vi "Supply Line Config.vi"(0 "Supply Line Handle in":refnum<k15>, 5 "SMU Config":T1={"Output Function"=1006, "Channel(s)"="", "Voltage Level"=0.0, "Current Level"=0.0, "Voltage Limit"=0.0, "Current Limit"=0.0, "Transient Response (V):Gain Bandwidth"=0.0, "Transient Response (V):Compensation Frequency"=0.0, "Transient Response (V):Pole-Zero Ratio"=0.0, "Transient Response"=1039, "Sense"=1009, "Transient Response (I):Gain Bandwidth"=0.0, "Transient Response (I):Compensation Frequency"=0.0, "Transient Response (I):Pole-Zero Ratio"=0.0} {"Sense" items=["Local"=1008, "Remote"=1009]; "Transient Response" items=["Slow"=1041, "Normal"=1038, "Fast"=1039, "Custom"=1042]; "output function" items=["DC Voltage"=1006, "DC Current"=1007, "Pulse Voltage"=1049, "Pulse Current"=1050]}, 11 "error in (no error)":errorcluster) -> (4 "Supply Line Handle out":refnum<k15>, 15 "error out":errorcluster)   [LabVIEW 2016, in "SMU.lvlib"]
uses:
  SMU.lvlib
  <instrlib>/niDCPower/nidcpower.llb/niDCPower Source Mode.ctl
  <instrlib>/niDCPower/nidcpower.llb/niDCPower Output Function.ctl
  Typedefs/Supply Line Configuration.ctl
panel:
  out "Source:Custom Transient Response:Current:Gain Bandwidth":dbl
  out "Source:Custom Transient Response:Current:Compensation Frequency":dbl
  out "Source:Custom Transient Response:Current:Pole-Zero Ratio":dbl
  out "Source:Custom Transient Response:Voltage:Pole-Zero Ratio":dbl
  out "Source:Custom Transient Response:Voltage:Compensation Frequency":dbl
  out "Source:Custom Transient Response:Voltage:Gain Bandwidth":dbl
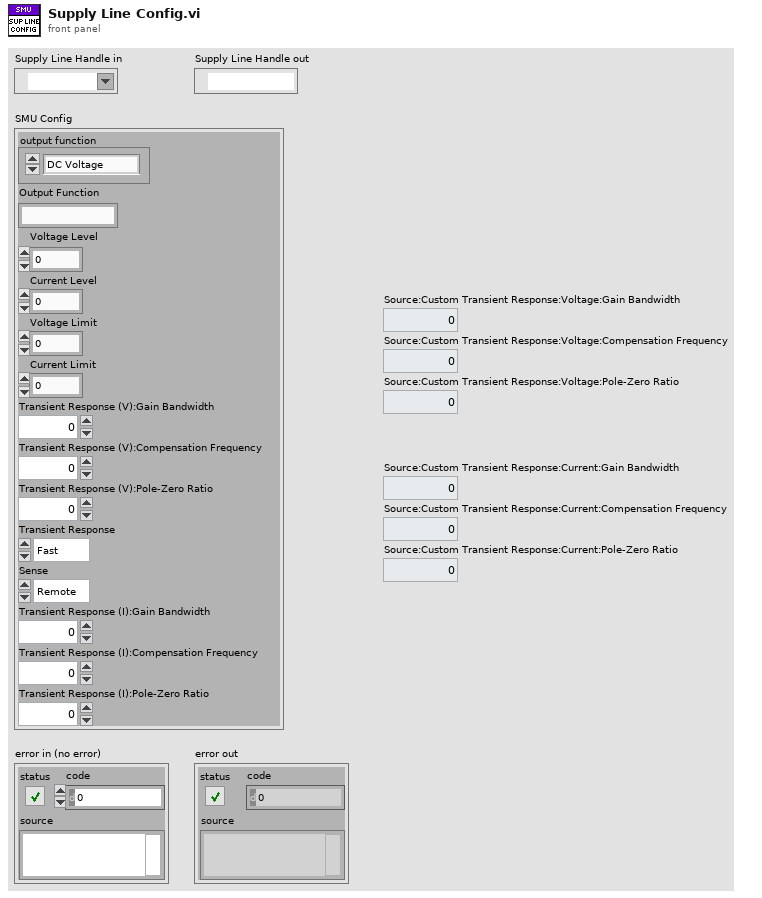
[diagram p1: front panel]
types:
  T1 = typedef "SMU.lvlib/Supply Line Configuration.ctl" = cluster{"Output Function":T2, "Channel(s)":string, "Voltage Level":dbl, "Current Level":dbl, "Voltage Limit":dbl, "Current Limit":dbl, "Transient Response (V):Gain Bandwidth":dbl, "Transient Response (V):Compensation Frequency":dbl, "Transient Response (V):Pole-Zero Ratio":dbl, "Transient Response":i32, "Sense":i32, "Transient Response (I):Gain Bandwidth":dbl, "Transient Response (I):Compensation Frequency":dbl, "Transient Response (I):Pole-Zero Ratio":dbl}
  T2 = typedef "niDCPower Output Function.ctl" = i32
  T3 = typedef "niDCPower Source Mode.ctl" = i32
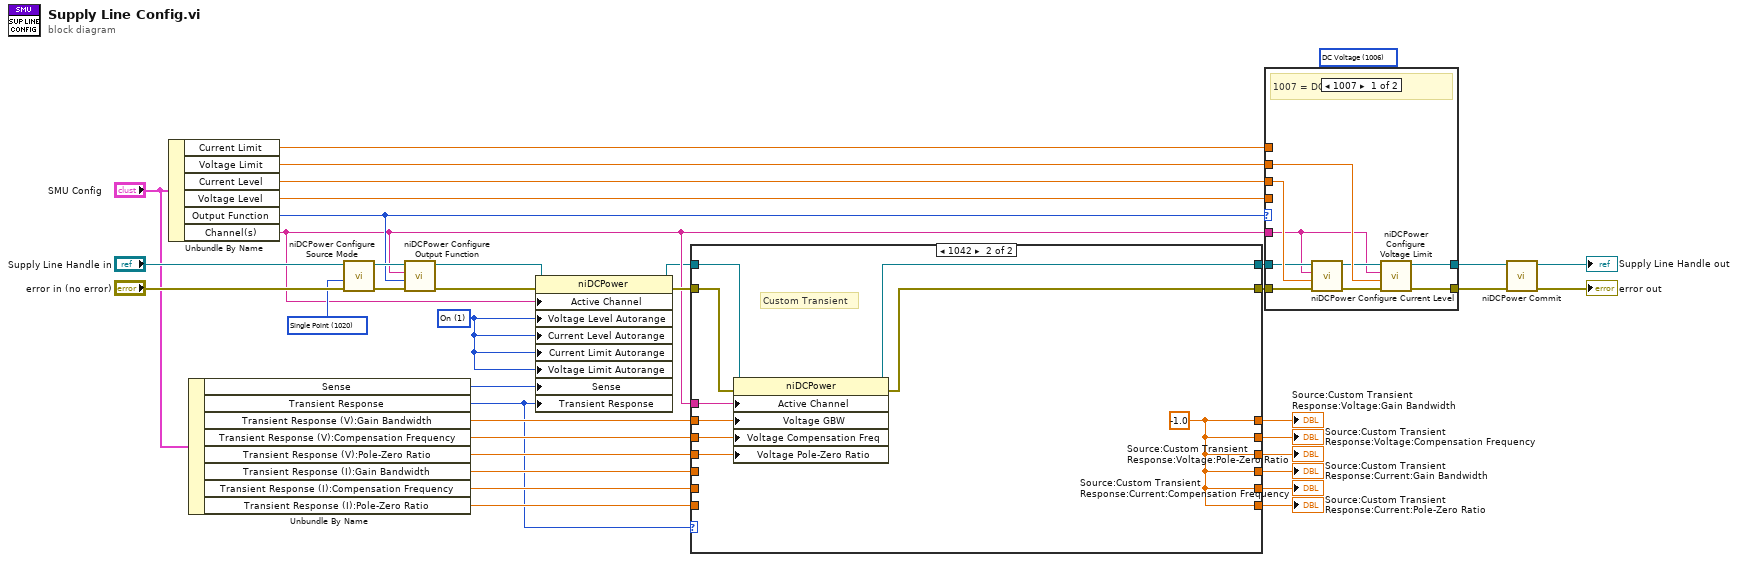
[diagram p0: block diagram]
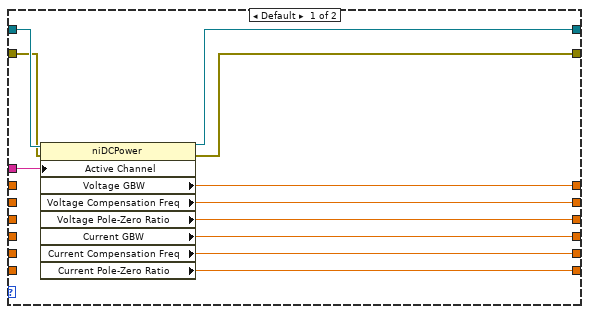
[diagram p2: hidden frame]
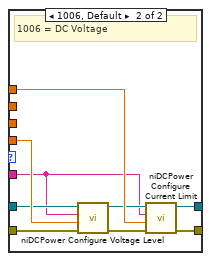
[diagram p3: hidden frame]
diagram:
  w20 = 1 items=["Off", "On"] ("Source:DC Voltage:Voltage Level Autorange")
  (unwired) T2 1006 items=["DC Voltage"=1006, "DC Current"=1007, "Pulse Voltage"=1049, "Pulse Current"=1050] ("Output Function")
  w31 = T3 1020 items=["Single Point"=1020, "Sequence"=1021] ("source mode")
  n1 = Unbundle By Name("SMU Config") -> ("Current Limit"=w28:dbl, "Voltage Limit"=w27:dbl, "Current Level"=w29:dbl, "Voltage Level"=w30:dbl, "Output Function"=w24:T2, "Channel(s)"=w17:string)
  n2 = Unbundle By Name("SMU Config") -> ("Sense"=w18:i32, "Transient Response"=w7:i32, "Transient Response (V):Gain Bandwidth"=w8:dbl, "Transient Response (V):Compensation Frequency"=w9:dbl, "Transient Response (V):Pole-Zero Ratio"=w10:dbl, "Transient Response (I):Gain Bandwidth"=w11:dbl, "Transient Response (I):Compensation Frequency"=w12:dbl, "Transient Response (I):Pole-Zero Ratio"=w13:dbl)
  n3 = call <instrlib>:"niDCPower Configure Source Mode.vi"("error in (no error)"="error in (no error)", "source mode"=w31, "instrument handle"="Supply Line Handle in") -> ("error out"=w37:errorcluster, "instrument handle out"=w25:refnum<k15>)  [unwired: 7 out]
  n4 = call <instrlib>:"niDCPower Configure Output Function.vi"("error in (no error)"=w37, "output function"=w24, "channel name"=w17, "instrument handle"=w25) -> ("error out"=w35:errorcluster, "instrument handle out"=w23:refnum<k15>)  [unwired: 6 in]
  n5 = property class="niDCPower"(reference=w23, error in=w35, "Active Channel"=w17, "Voltage Level Autorange"=w20, "Current Level Autorange"=w20, "Current Limit Autorange"=w20, "Voltage Limit Autorange"=w20, "Sense"=w18, "Transient Response"=w7) -> (reference out=w14:refnum<k15>, error out=w32:errorcluster)
  n6 = case shown="1042" w7 {
    tunnel: w32 -> [w44 w57]
    tunnel: w17 -> [w48 w56]
    tunnel: [w46 w55] -> w16
    tunnel: [w45 w54] -> w15
    tunnel: w14 -> [w47 w53]
    tunnel: w13 -> [_ _]
    tunnel: w12 -> [_ _]
    tunnel: w11 -> [_ _]
    tunnel: w10 -> [_ w52]
    tunnel: w9 -> [_ w51]
    tunnel: w8 -> [_ w50]
    tunnel: [w43 w49] -> w6
    tunnel: [w42 w49] -> w5
    tunnel: [w41 w49] -> w4
    tunnel: [w40 w49] -> w3
    tunnel: [w39 w49] -> w2
    tunnel: [w38 w49] -> w1
    frame Default {
      n7 = property class="niDCPower"(reference=w47, error in=w44, "Active Channel"=w48) -> (reference out=w46:refnum<k15>, error out=w45:errorcluster, "Voltage GBW"=w43:dbl, "Voltage Compensation Freq"=w42:dbl, "Voltage Pole-Zero Ratio"=w41:dbl, "Current GBW"=w40:dbl, "Current Compensation Freq"=w39:dbl, "Current Pole-Zero Ratio"=w38:dbl)
    }
    frame 1042 {
      w49 = -1.0 ("Voltage GBW")
      # "Custom Transient"
      n8 = property class="niDCPower"(reference=w53, error in=w57, "Active Channel"=w56, "Voltage GBW"=w50, "Voltage Compensation Freq"=w51, "Voltage Pole-Zero Ratio"=w52) -> (reference out=w55:refnum<k15>, error out=w54:errorcluster)
    }
  }
  "Source:Custom Transient Response:Voltage:Gain Bandwidth" <- w6
  "Source:Custom Transient Response:Voltage:Compensation Frequency" <- w5
  "Source:Custom Transient Response:Voltage:Pole-Zero Ratio" <- w4
  "Source:Custom Transient Response:Current:Gain Bandwidth" <- w3
  "Source:Custom Transient Response:Current:Compensation Frequency" <- w2
  "Source:Custom Transient Response:Current:Pole-Zero Ratio" <- w1
  n9 = case shown="1007" w24 {
    tunnel: [w63 w72] -> w22
    tunnel: w17 -> [w58 w67]
    tunnel: w30 -> [_ w71]
    tunnel: w29 -> [w62 _]
    tunnel: w28 -> [_ w70]
    tunnel: w27 -> [w61 _]
    tunnel: [w65 w74] -> w34
    tunnel: w16 -> [w59 w68]
    tunnel: w15 -> [w64 w73]
    frame 1007 {
      # "1007 = DC Current"
      n10 = call <instrlib>:"niDCPower Configure Current Level.vi"("error in (no error)"=w64, "current level"=w62, "channel name"=w58, "instrument handle"=w59) -> ("error out"=w66:errorcluster, "instrument handle out"=w60:refnum<k15>)  [unwired: 6 in]
      n11 = call <instrlib>:"niDCPower Configure Voltage Limit.vi"("error in (no error)"=w66, "voltage limit"=w61, "channel name"=w58, "instrument handle"=w60) -> ("error out"=w65:errorcluster, "instrument handle out"=w63:refnum<k15>)  [unwired: 6 in]
    }
    frame 1006, Default {
      # "1006 = DC Voltage"
      n12 = call <instrlib>:"niDCPower Configure Voltage Level.vi"("error in (no error)"=w73, "voltage level"=w71, "channel name"=w67, "instrument handle"=w68) -> ("error out"=w75:errorcluster, "instrument handle out"=w69:refnum<k15>)  [unwired: 6 out]
      n13 = call <instrlib>:"niDCPower Configure Current Limit.vi"("error in (no error)"=w75, "current limit"=w70, "channel name"=w67, "instrument handle"=w69) -> ("error out"=w74:errorcluster, "instrument handle out"=w72:refnum<k15>)  [unwired: 1 in, 5 out]
    }
  }
  n14 = call <instrlib>:"niDCPower Commit.vi"("error in (no error)"=w34, "instrument handle"=w22) -> ("error out"=→"error out":errorcluster, "instrument handle out"=→"Supply Line Handle out":refnum<k15>)  [unwired: 8 in]
